vi "SRS SIM 900 Modules.vi"(1 "Action":T6=enum."Identify", 2 "Parameters":variant) -> (6 "Output":variant, 7 "Stop":bool)   [LabVIEW 2019]
uses:
  Sub Controls/Instrument Actions.ctl
  Sub Controls/Public.ctl
  Sub Controls/Instrument Match.ctl
  SubVIs/SIM 921 Options.ctl
  Sub Controls/Factory Reset.ctl
  Sub Controls/Scan Output.ctl
  Sub Controls/Instrument IDN.ctl
  Sub Controls/User Event Command.ctl
  <vilib>/Instr/_visa.llb/VISA GPIB Control REN Mode.ctl
panel:
  in  "Factory Reset":T1
  out "Channel Index":i32
  in  "Values Returned":T2={"X"=TRUE, "X&Y"=FALSE, "R"=FALSE, "R & ϴ"=FALSE}
  in  "SIM Slot #":T3(radio)
  out "Title":string="Stanford Research Small Instrument Modules"
  in  "VISA resource name":refnum<visa-resource-name>
  in  "Instruments":T4[](array[typedef])=[{"Model"="SIM921", "Manufacturer"="Stanford_Research_Systems", "Term Character"="", "Wait Time (mS)"=0, "Wait for SRQ"=FALSE, "Type"="AC Resistance"}]
  out "Model":string
  in  "Address":u16(ring)
  in  "Public":T5
  out "Measurement":dbl[](array[numeric]) format="%^.3e"
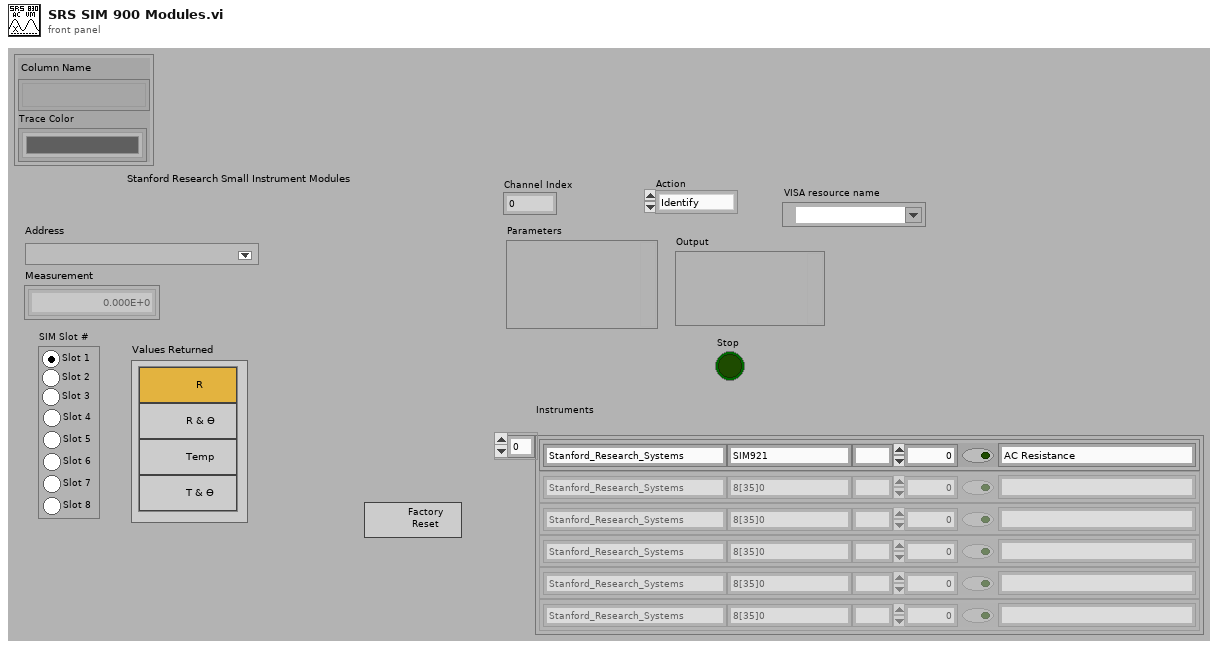
[diagram p1: front panel]
types:
  T1 = typedef "Factory Reset.ctl" = bool
  T2 = typedef "SIM 921 Options.ctl" = cluster{"X":bool, "X&Y":bool, "R":bool, "R & ϴ":bool}
  T3 = enum32{"Slot 1", "Slot 2", "Slot 3", "Slot 4", "Slot 5", "Slot 6", "Slot 7", "Slot 8"}
  T4 = typedef "Instrument Match.ctl" = cluster{"Model":string, "Manufacturer":string, "Term Character":string, "Wait Time (mS)":u32, "Wait for SRQ":bool, "Type":string}
  T5 = typedef "Public.ctl" = cluster{"Column Name":string[], "Trace Color":u32[]}
  T6 = typedef "Instrument Actions.ctl" = enum16{"Scan", "Identify", "New", "Configure", "Initialize", "Test", "Read", "Close"}
  T7 = typedef "Scan Output.ctl" = cluster{"Manufacturer":string, "Model":string, "Info":string, "Revision":string, "error out":errorcluster}
  T8 = typedef "Instrument IDN.ctl" = cluster{"VISA Address":string, "Status":u16, "Manufacturer":string, "Model":string, "Info":string, "Info 2":string, "Misc Data":variant}
  T9 = enum8{"Enabled", "Disabled", "Disabled and Grayed Out"}
  T10 = typedef "User Event Command.ctl" = enum32{"Stop Config"}
  T11 = typedef "VISA GPIB Control REN Mode.ctl" = u16
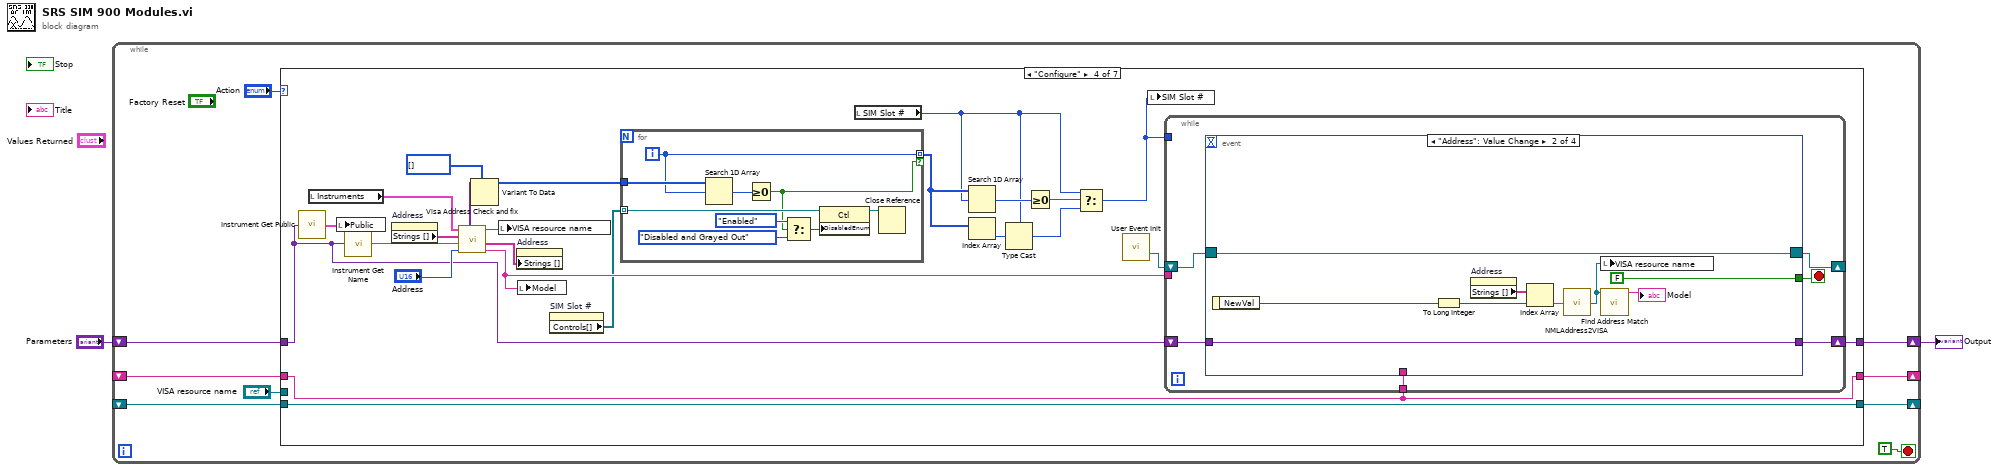
[diagram p0: block diagram]
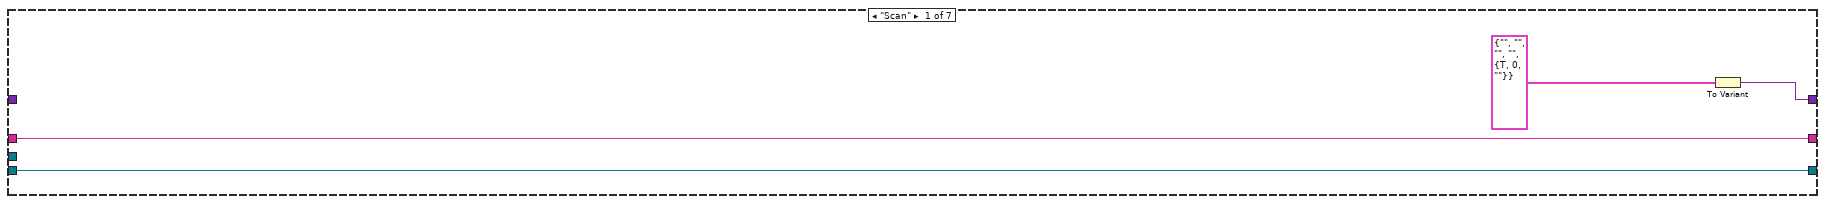
[diagram p2: hidden frame]
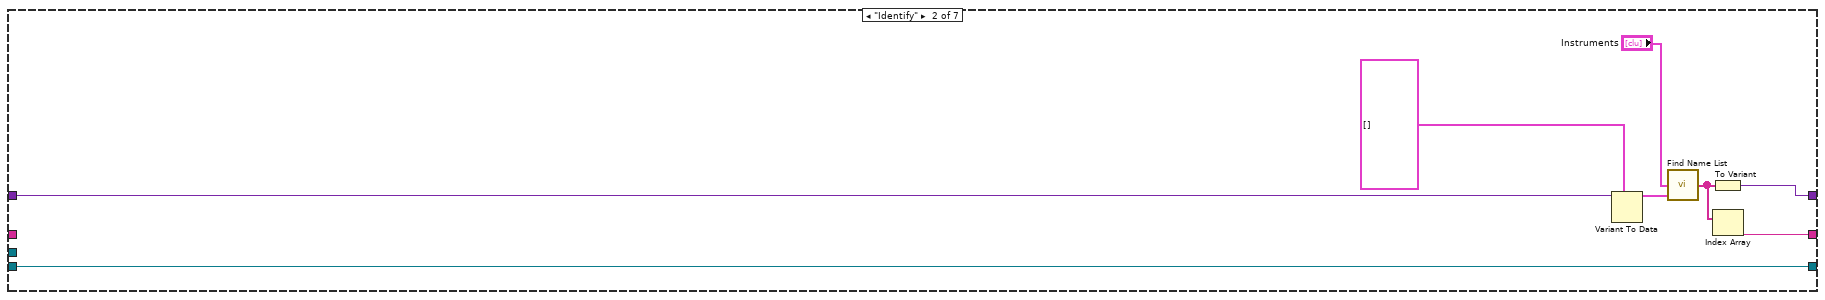
[diagram p3: hidden frame]
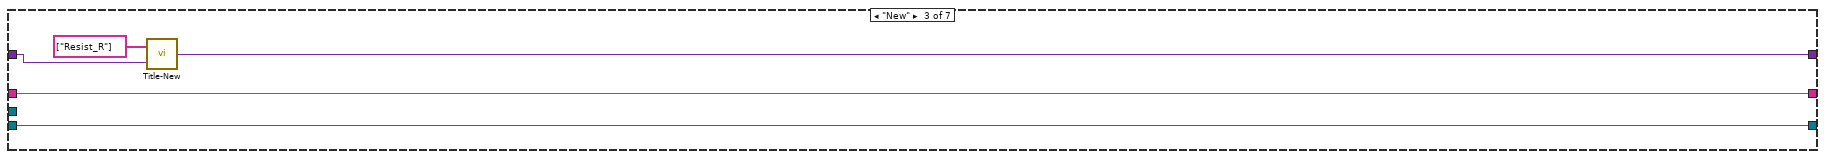
[diagram p4: hidden frame]
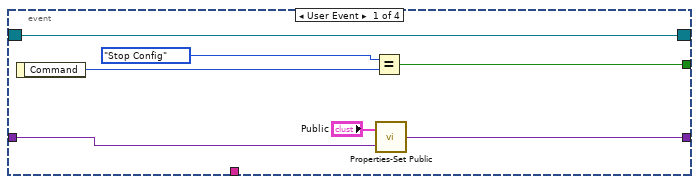
[diagram p5: hidden frame]
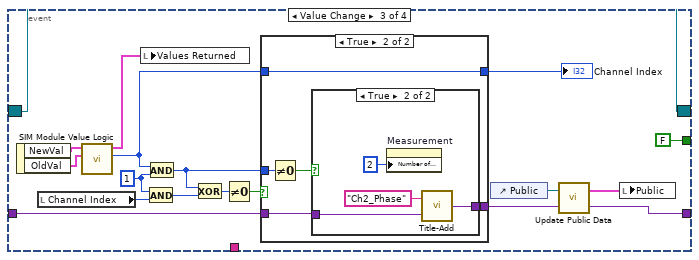
[diagram p6: hidden frame]
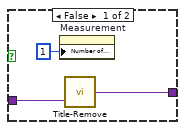
[diagram p8: hidden frame]
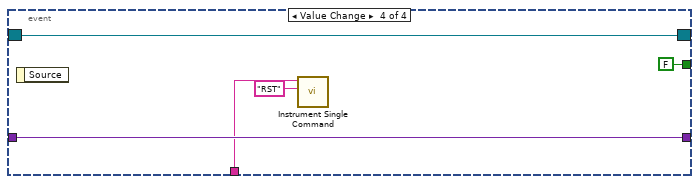
[diagram p9: hidden frame]
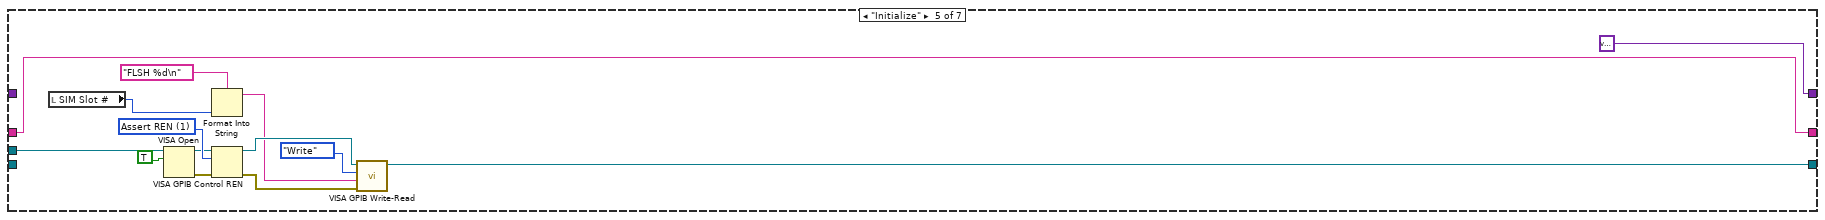
[diagram p10: hidden frame]
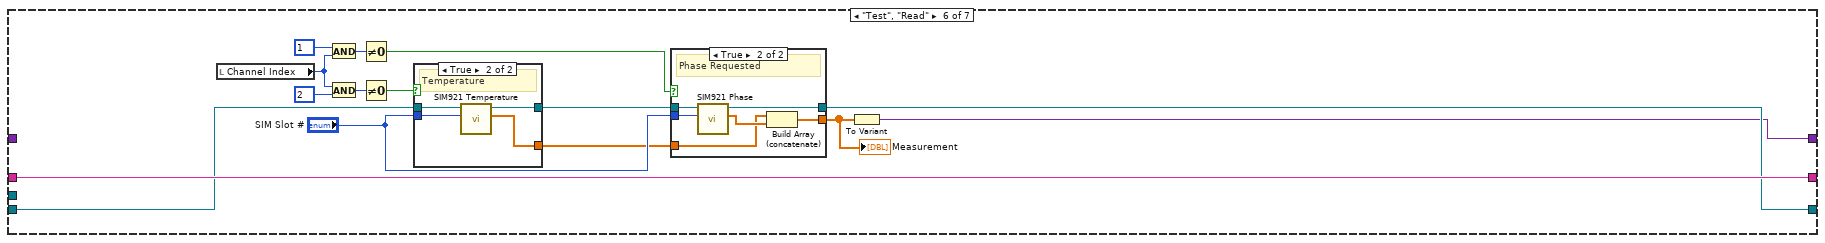
[diagram p11: hidden frame]
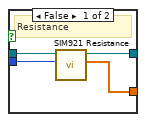
[diagram p12: hidden frame]
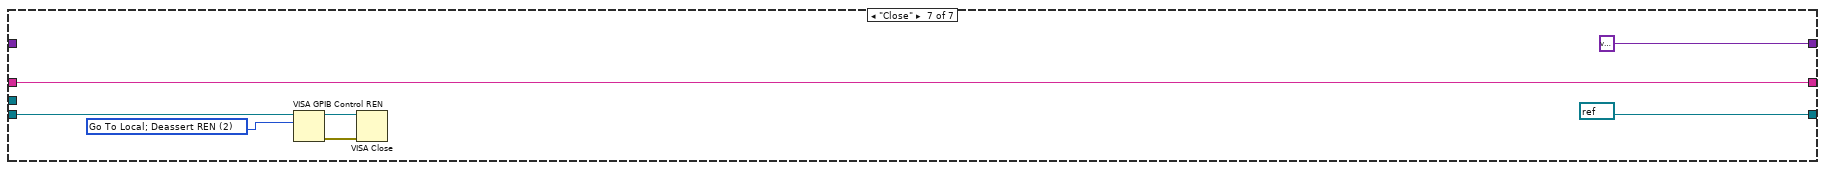
[diagram p14: hidden frame]
diagram:
  n1 = while {
    shift-right: [w10] -> _
    shift-left: _ -> [w9]
    shift-right: [w7] -> w1
    shift-left: "Parameters" -> [w8]
    shift-right: [w4] -> _
    shift-left: _ -> [w3]
    stop <- TRUE stop-if-true
    n2 = case shown="\"Configure\"" "Action" {
      tunnel: [w14 w23 w27 w52 w126 w146 refnum<visa-resource-name> refnum ("Open VISA Resource name")] -> w10
      tunnel: w9 -> [w14 w23 w27 w52 _ w148 w167]
      tunnel: w8 -> [_ w20 w28 w42 _ _ _]
      tunnel: [w13 w22 w25 w51 variant ("Variant") w143 variant ("Variant")] -> w7
      tunnel: "VISA resource name" -> [_ _ _ _ w129 _ _]
      tunnel: [w12 w16 w24 w29 w128 w149 w166] -> w4
      tunnel: w3 -> [w12 _ w24 w29 w128 w149 w166]
      frame "Scan" {
        n3 = To Variant(anything=T7 {"Manufacturer"="", "Model"="", "Info"="", "Revision"="", "error out"={"status"=TRUE, "code"=0, "source"=""}} ("Scan Output")) -> (Variant=w13:variant)
      }
      frame "Identify" {
        n4 = Variant To Data(type=T8[] [], Variant=w20) -> (data=w18:T8[])  [unwired: 1 in, 1 out]
        n5 = call "Find Name List.vi"("Bus Scan"=w18, "Instruments"="Instruments") -> ("Names"=w17:string[])  [unwired: 1 in]
        n6 = To Variant(anything=w17) -> (Variant=w22:variant)
        n7 = Index Array(array=w17) -> (element=w16:string)  [unwired: 1 in]
      }
      frame "New" {
        n8 = call "Title-New.vi"("Parameters"=w28, "Array"=string[] ["Resist_R"]) -> ("Instrument Prop"=w25:variant)
      }
      frame "Configure" {
        n9 = call "Instrument Get Public.vi"("Variant"=w42) -> ("Public"=w50:T5)
        n10 = local read "Instruments"() -> (w41:T4[])
        n11 = local write "Public"(w50) -> ()
        n12 = call "Instrument Get Name.vi"("Parameters"=w42) -> ("Type"=w43:string)
        n13 = property on="Address" class="Ring (strict)"() -> ("Strings []"=w47:string[])  [unwired: 2 in, 2 out]
        n14 = call "Visa Address Check and fix.vi"("Address"="Address", "Name"=w43, "NML Addresses"=w47, "Instruments"=w41) -> ("Model"=w44:string, "NML Addresses"=w45:string[], "VISA resource name"=w46:refnum<visa-resource-name>, "Array"=w39:variant[])  [unwired: 2 out]
        n15 = Variant To Data(type=i32[] [], Variant=w39) -> (data=w38:i32[])  [unwired: 1 in, 1 out]
        n16 = local write "VISA resource name"(w46) -> ()
        n17 = property on="Address" class="Ring (strict)"("Strings []"=w45) -> ()  [unwired: 2 in, 2 out]
        n18 = local write "Model"(w44) -> ()
        n19 = property on="SIM Slot #" class="RadioBtnsControl (strict)"() -> ("Controls[]"=w37:refnum<vi>[])  [unwired: 2 in, 2 out]
        n20 = for {
          tunnel: w37 -> [w59] mode=indexing
          tunnel: w38 -> [w61]
          tunnel: [w54] -> w36 mode=indexing if=w53
          i -> [w54]
          n21 = Search 1D Array(1D array=w61, element=w54) -> (index of element=w60:i32)  [unwired: 1 in]
          n22 = Greater Or Equal To 0?(x=w60) -> (x >= 0?=w53:bool)
          n23 = Select(t=T9."Enabled" ("Disabled"), s=w53, f=T9."Disabled and Grayed Out" ("Disabled")) -> (s? t:f=w56:T9)
          n24 = property class="Ctl"(reference=w59, "DisabledEnum"=w56) -> (reference out=w58:refnum<vi>)  [unwired: 1 in, 1 out]
          n25 = Close Reference(reference=w58) -> ()  [unwired: 1 in, 1 out]
        }
        n26 = local read "SIM Slot #"() -> (w30:T3)
        n27 = Search 1D Array(1D array=w36, element=w30) -> (index of element=w35:i32)  [unwired: 1 in]
        n28 = Index Array(array=w36) -> (element=w33:i32)  [unwired: 1 in]
        n29 = Type Cast(type=w30, x=w33) -> (*(type *) &x=w32:T3)
        n30 = Greater Or Equal To 0?(x=w35) -> (x >= 0?=w34:bool)
        n31 = Select(t=w30, s=w34, f=w32) -> (s? t:f=w31:T3)
        n32 = call "User Event Init.vi"() -> ("Event Registration Refnum"=w49:refnum<event-registration>)  [unwired: 14 in, 1 out]
        n33 = local write "SIM Slot #"(w31) -> ()
        n34 = while {
          shift-right: [w67] -> w51
          shift-left: w42 -> [w66]
          shift-right: [w63] -> _
          shift-left: w49 -> [w64]
          tunnel: w44 -> [_]
          tunnel: w31 -> [_]
          tunnel: w29 -> [w62]
          stop <- w65 stop-if-true
          n35 = event shown="[1] \"Address\": Value Change" {
            selector: w64 -> [w68 w83 w100 w118]
            dyn-events: [w68 w83 w100 w118] -> w63
            timeout: _ -> [_ _ _ _]
            tunnel: [w70 FALSE FALSE FALSE] -> w65
            tunnel: w66 -> [w73 w77 w95 w119]
            tunnel: [w74 w77 w97 w119] -> w67
            tunnel: w62 -> [_ _ _ w116]
            event User Event {
              n36 = event-data() -> ("Command"=w72:T10)  [unwired: 1 in]
              n37 = Equal?(x=User_Event_Command."Stop Config", y=w72) -> (x = y?=w70:bool)
              n38 = call "Properties-Set Public.vi"("Variant"=w73, "New Public"="Public") -> ("Variant 2"=w74:variant)
            }
            event "Address": Value Change {
              n39 = event-data() -> ("NewVal"=w81:u16)  [unwired: 1 in]
              n40 = To Long Integer(number=w81) -> (32bit integer=w75:i32)
              n41 = property on="Address" class="Ring (strict)"() -> ("Strings []"=w80:string[])  [unwired: 2 in, 2 out]
              n42 = Index Array(array=w80, index=w75) -> (element=w79:string)
              n43 = call "NMLAddress2VISA.vi"("NML Address"=w79) -> ("VISA resource name"=w76:refnum<visa-resource-name>)
              n44 = local write "VISA resource name"(w76) -> ()
              n45 = call "Find Address Match.vi"("VISA resource name"=w76) -> ("Model"=→"Model":string)  [unwired: 3 in, 3 out]
            }
            event Value Change {
              w88 = 1 ("y")
              n46 = event-data() -> ("NewVal"=w94:T2, "OldVal"=w93:T2)  [unwired: 1 in]
              n47 = local read "Channel Index"() -> (w91:i32)
              n48 = call "SIM Module Value Logic.vi"("Old Channels"=w93, "New Channels"=w94) -> ("index of element"=w85:i32, "Channels Out"=w92:T2)  [unwired: 8 in]
              n49 = local write "Values Returned"(w92) -> ()
              n50 = And(x=w88, y=w91) -> (x .and. y?=w89:i32)
              n51 = And(x=w85, y=w88) -> (x .and. y?=w86:i32)
              n52 = Exclusive Or(1:w89, 2:w86) -> (0:w90:i32)
              n53 = Not Equal To 0?(x=w90) -> (x != 0?=w87:bool)
              n54 = case shown="True" w87 {
                tunnel: [w103 w108] -> w99
                tunnel: w95 -> [w103 w107]
                tunnel: w86 -> [_ w106]
                tunnel: w85 -> [w102 w104]
                tunnel: [w102 w104] -> w84
                frame False {
                }
                frame True {
                  n55 = Not Equal To 0?(x=w106) -> (x != 0?=w105:bool)
                  n56 = case shown="True" w105 {
                    tunnel: w107 -> [w109 w112]
                    tunnel: [w111 w115] -> w108
                    frame False {
                      n57 = property on="Measurement" class="Arr (strict)"("Number of Columns"=u32 1) -> ()  [unwired: 2 in, 2 out]
                      n58 = call "Title-Remove.vi"("Parameters"=w109) -> ("Variant"=w111:variant)  [unwired: 1 in]
                    }
                    frame True {
                      n59 = property on="Measurement" class="Arr (strict)"("Number of Columns"=u32 2) -> ()  [unwired: 2 in, 2 out]
                      n60 = call "Title-Add.vi"("Parameters"=w112, "String"="Ch2_Phase") -> ("Variant"=w115:variant)
                    }
                  }
                }
              }
              "Channel Index" <- w84
              n61 = control-ref of="Public"() -> (w98:refnum<vi>)
              n62 = call "Update Public Data.vi"("Variant In"=w99, "Public 2"=w98) -> ("Variant Out"=w97:variant, "Public"=w96:T5)
              n63 = local write "Public"(w96) -> ()
            }
            event Value Change {
              n64 = event-data() -> ()  [unwired: 1 in, 1 out]
              n65 = call "Instrument Single Command.vi"("Reset Command"="RST", "VISA Name"=w116) -> ()  [unwired: 9 in, 1 out]
            }
          }
        }
      }
      frame "Initialize" {
        w133 = T11 1 items=["Deassert REN", "Assert REN", "Go To Local; Deassert REN ", "Assert REN; Address Device", "Local Lockout (Addressed Devices)", "Local Lockout (This Device)", "Go To Local"] ("Mode")
        n66 = local read "SIM Slot #"() -> (w122:T3)
        n67 = VISA Open(duplicate session (F)=TRUE, VISA resource name=w129) -> (VISA resource name=w131:refnum<visa-resource-name>, error out=w132:errorcluster)  [unwired: 3 in]
        n68 = Format Into String(format string="FLSH %d\n", w122) -> (resulting string=w121:string)  [unwired: 2 in, 1 out]
        n69 = VISA GPIB Control REN(8:w132, 10:w133, 11:w131) -> (0:w125:errorcluster, 3:w127:refnum<visa-resource-name>)
        n70 = call "VISA GPIB Write-Read.vi"("error in (no error)"=w125, "Command"=w121, "Action"=enum16{"Write", "Read", "Write & Read"}."Write", "VISA resource name"=w127) -> ("dup VISA Session"=w126:refnum<visa-resource-name>)  [unwired: 4 in, 3 out]
      }
      frame "Test", "Read" {
        n71 = local read "Channel Index"() -> (w142:i32)
        n72 = And(x=1, y=w142) -> (x .and. y?=w139:i32)
        n73 = And(x=w142, y=2 ("x")) -> (x .and. y?=w138:i32)
        n74 = Not Equal To 0?(x=w139) -> (x != 0?=w137:bool)
        n75 = Not Equal To 0?(x=w138) -> (x != 0?=w136:bool)
        n76 = case shown="True" w136 {
          tunnel: w148 -> [w153 w157]
          tunnel: [w152 w156] -> w147
          tunnel: "SIM Slot #" -> [w151 w155]
          tunnel: [w150 w154] -> w144
          frame False {
            # "Resistance"
            n77 = call "SIM921 Resistance.vi"("Slot"=w151, "VISA resource name"=w153) -> ("Resistance"=w150:dbl[], "VISA resource name"=w152:refnum<visa-resource-name>)  [unwired: 8 in]
          }
          frame True {
            # "Temperature"
            n78 = call "SIM921 Temperature.vi"("Slot"=w155, "VISA resource name"=w157) -> ("Temperature"=w154:dbl[], "VISA resource name"=w156:refnum<visa-resource-name>)  [unwired: 8 in]
          }
        }
        n79 = case shown="True" w137 {
          tunnel: [w158 w160] -> w135
          tunnel: w147 -> [w159 w165]
          tunnel: [w159 w163] -> w146
          tunnel: "SIM Slot #" -> [_ w164]
          tunnel: w144 -> [w158 w161]
          frame False {
          }
          frame True {
            # "Phase Requested"
            n80 = call "SIM921 Phase.vi"("Slot"=w164, "VISA resource name"=w165) -> ("Resistance"=w162:dbl[], "VISA resource name"=w163:refnum<visa-resource-name>)  [unwired: 8 in]
            n81 = Build Array (concatenate)(w161, w162) -> (w160:dbl[])
          }
        }
        "Measurement" <- w135
        n82 = To Variant(anything=w135) -> (Variant=w143:variant)
      }
      frame "Close" {
        w171 = T11 2 items=["Deassert REN", "Assert REN", "Go To Local; Deassert REN ", "Assert REN; Address Device", "Local Lockout (Addressed Devices)", "Local Lockout (This Device)", "Go To Local"] ("Mode")
        n83 = VISA GPIB Control REN(10:w171, 11:w167) -> (0:w170:errorcluster, 3:w169:refnum<visa-resource-name>)  [unwired: 1 in]
        n84 = VISA Close(VISA resource name=w169, error in (no error)=w170) -> ()  [unwired: 1 out]
      }
    }
  }
  "Output" <- w1
